vi "Create Thermocouple Channel.vi"(6 "index":i32, 7 "thermocouple channel settings":T1={"thermocouple type"=enum."J", "measurement units"=enum."Degrees Celsius"}, 8 "error in":errorcluster, 9 "default value":dbl, 10 "name":string, 11 "thermocouple channel in":refnum<class "Thermocouple Channel.lvclass">) -> (0 "error out":errorcluster, 3 "thermocouple channel out":refnum<class "Thermocouple Channel.lvclass">)   [LabVIEW 2020, in "Scan Engine Scripting.lvlib" / "Thermocouple Channel.lvclass"]
uses:
  Thermocouple Channel.lvclass
  Thermocouple Channel Settings.ctl
  Thermocouple Type.ctl
  Measurement Units.ctl
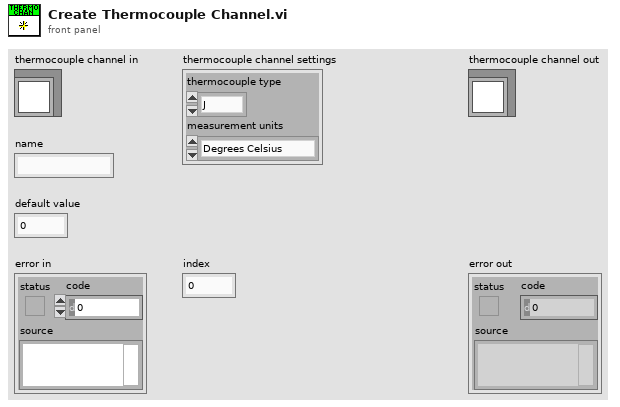
[diagram p1: front panel]
types:
  T1 = typedef "Scan Engine Scripting.lvlib/Thermocouple Channel.lvclass/Thermocouple Channel Settings.ctl" = cluster{"thermocouple type":T2, "measurement units":T3}
  T2 = typedef "Scan Engine Scripting.lvlib/Thermocouple Channel.lvclass/Thermocouple Type.ctl" = enum16{"J", "K", "T", "E", "R", "S", "N", "B"}
  T3 = typedef "Scan Engine Scripting.lvlib/Thermocouple Channel.lvclass/Measurement Units.ctl" = enum16{"Raw Volts", "Degrees Kelvin", "Degrees Celsius", "Degrees Fahrenheit", "Degrees Rankine"}
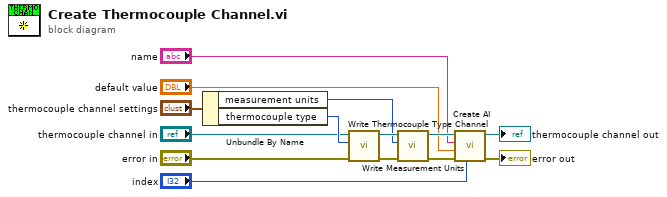
[diagram p0: block diagram]
diagram:
  n1 = Unbundle By Name("thermocouple channel settings") -> ("measurement units"=w10:T3, "thermocouple type"=w13:T2)
  n2 = call-dynamic "Write Thermocouple Type.vi"("error in"="error in", "thermocouple type"=w13, "thermocouple channel in"="thermocouple channel in") -> ("error out"=w9:errorcluster, "thermocouple channel out"=w11:refnum<class "Thermocouple Channel.lvclass">)  [unwired: 7 in]
  n3 = call-dynamic "Write Measurement Units.vi"("error in"=w9, "measurement units"=w10, "thermocouple channel in"=w11) -> ("error out"=w8:errorcluster, "thermocouple channel out"=w7:refnum<class "Thermocouple Channel.lvclass">)  [unwired: 7 in]
  n4 = call-dynamic "Create AI Channel.vi"("index"="index", "error in"=w8, "default value"="default value", "name"="name", "AI channel in"=w7) -> ("error out"=→"error out":errorcluster, "AI channel out"=→"thermocouple channel out":refnum<class "Thermocouple Channel.lvclass">)  [unwired: 5 in]
